vi "Read EXT.vi"(8 "error in (no error)":errorcluster, 11 "Local Bus in":refnum<class "Local Bus.lvclass">) -> (0 "error out":errorcluster, 2 "EXT":refnum<data-value>, 3 "Local Bus out":refnum<class "Local Bus.lvclass">)   [LabVIEW 2021, in "Local Bus.lvclass"]
uses:
  Local Bus.lvclass
  Local Bus.lvclass/Local Bus.ctl
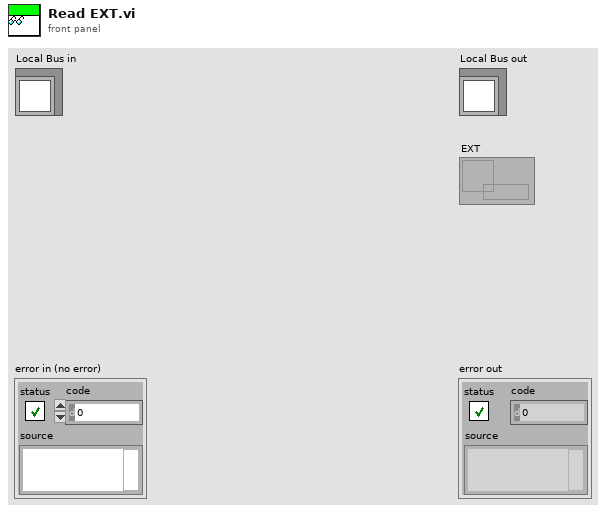
[diagram p1: front panel]
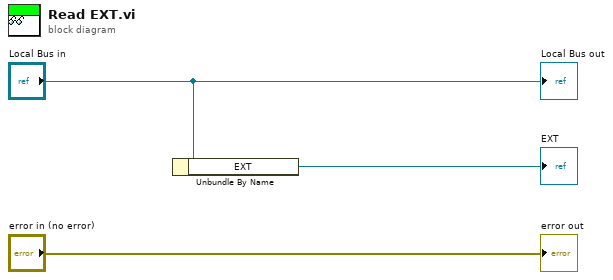
[diagram p0: block diagram]
diagram:
  n1 = Unbundle By Name("Local Bus in") -> ("EXT"=→"EXT":refnum<data-value>)
  "error out" <- "error in (no error)"
  "Local Bus out" <- "Local Bus in"
